vi "Configure Tracking.vi"(7 "Enable Tracking (F: False)":bool, 8 "error in (no error)":errorcluster, 11 "VISA resource name":refnum<visa-resource-name>) -> (0 "error out":errorcluster, 3 "VISA resource name out":refnum<visa-resource-name>)   [LabVIEW 2010, in "Agilent E363X Series.lvlib"]
doc: "Enables or disables the power supply to operate in the track mode. When tracking mode is enabled, the +/-25V channels will have equal but opposite voltage levels.\n\n<B>Note:</B> Only supported on E3631"
uses:
  <instrlib>/Agilent E363X Series/Agilent E363X Series.lvlib
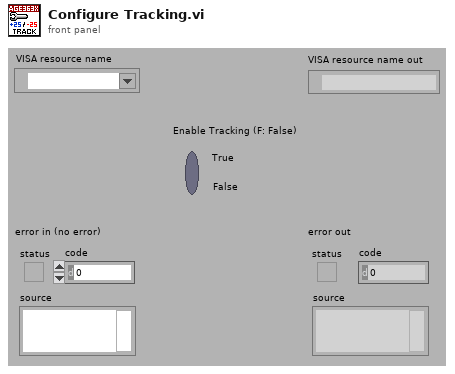
[diagram p1: front panel]
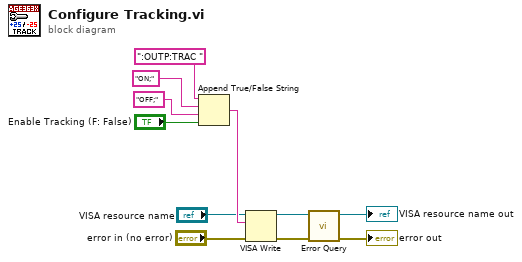
[diagram p0: block diagram]
diagram:
  n1 = Append True/False String(1:"Enable Tracking (F: False)", 2:"OFF;", 3:"ON;", 4:":OUTP:TRAC ") -> (0:w10:string)
  n2 = VISA Write(VISA resource name="VISA resource name", write buffer=w10, error in (no error)="error in (no error)") -> (VISA resource name out=w4:refnum<visa-resource-name>, error out=w3:errorcluster)  [unwired: 1 out]
  n3 = call <instrlib>:"Error Query.vi"("error in (no error)"=w3, "VISA resource name"=w4) -> ("error out"=→"error out":errorcluster, "VISA resource name out"=→"VISA resource name out":refnum<visa-resource-name>)  [unwired: 6 in, 2 out]
